vi "Pins to NI-DMM Sessions.vi"(8 "error in (no error)":errorcluster, 9 "Pins":string[](array[string]), 10 "Semiconductor Module Context":T1) -> (0 "error out":errorcluster, 1 "Channel Lists":string[](array[string]), 2 "Semiconductor Module Context Out":T1, 3 "Instrument Sessions":refnum<k15>[](array[refnum]), 5 "Pin Query Context":refnum<class "MultiplePinMultipleSessionQueryContext.lvclass">)   [LabVIEW 2013, in "DMM Custom Instruments.lvlib"]
uses:
  DMM Custom Instruments.lvlib
  <vilib>/NI_TestStand_SemiconductorModule/NI_TestStand_Semiconductor_Module.lvlibp/PinMap/General/SemiconductorModuleContext.ctl
  <vilib>/NI_TestStand_SemiconductorModule/NI_TestStand_Semiconductor_Module.lvlibp/PinMap/PinQueryContext/MultiplePinMultipleSessionQueryContext/MultiplePinMultipleSessionQueryContext.lvclass
  <vilib>/NI_TestStand_SemiconductorModule/NI_TestStand_Semiconductor_Module.lvlibp
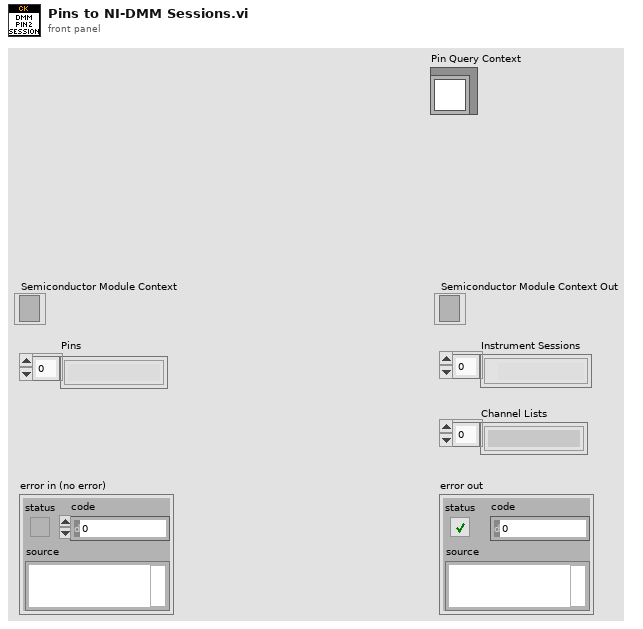
[diagram p1: front panel]
types:
  T1 = typedef "NI_TestStand_Semiconductor_Module.lvlibp/SemiconductorModuleContext.ctl" = refnum<k7>
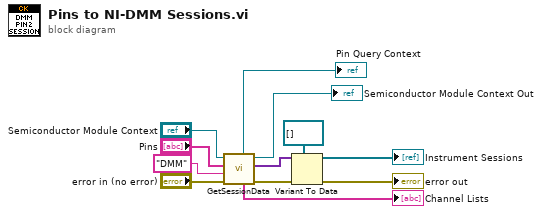
[diagram p0: block diagram]
diagram:
  n1 = call <vilib>:"GetSessionData.vi"("error in (no error)"="error in (no error)", "Instrument Type Id"="DMM", "Pins"="Pins", "Semiconductor Module Context"="Semiconductor Module Context") -> ("error out"=w7:errorcluster, "Session Data"=w6:variant[], "Semiconductor Module Context Out"=→"Semiconductor Module Context Out":T1, "Channel Lists"=→"Channel Lists":string[], "Pin Query Context"=→"Pin Query Context":refnum<class "MultiplePinMultipleSessionQueryContext.lvclass">)  [unwired: 2 in, 1 out]
  n2 = Variant To Data(error in=w7, type=refnum<k15>[] [], Variant=w6) -> (data=→"Instrument Sessions":refnum<k15>[], error out=→"error out":errorcluster)
